vi "GuardarColor.vi"(0 "NombreOperario":string, 3 "TokenColor":T1) -> (5 "HistorialDeColoresOutput":string[](array[string]), 6 "Total De Fichas":dbl, 7 "White":dbl, 9 "Blue":dbl, 10 "Red":dbl)   [LabVIEW 2017]
uses:
  Control/EnumControl.ctl
  Control/ColorTypeEnum.ctl
panel:
  out "Error":string
  out "Verificate2Times":bool
  out "Historial de colores":dbl[](array[numeric])
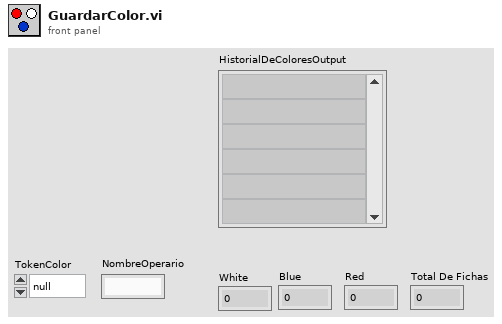
[diagram p1: front panel]
types:
  T1 = typedef "ColorTypeEnum.ctl" = enum16{"null", "White", "Blue", "Red"}
  T2 = typedef "EnumControl.ctl" = enum16{"Default", "Mostrar", "Guardar", "Reiniciar", "Stop", "Error"}
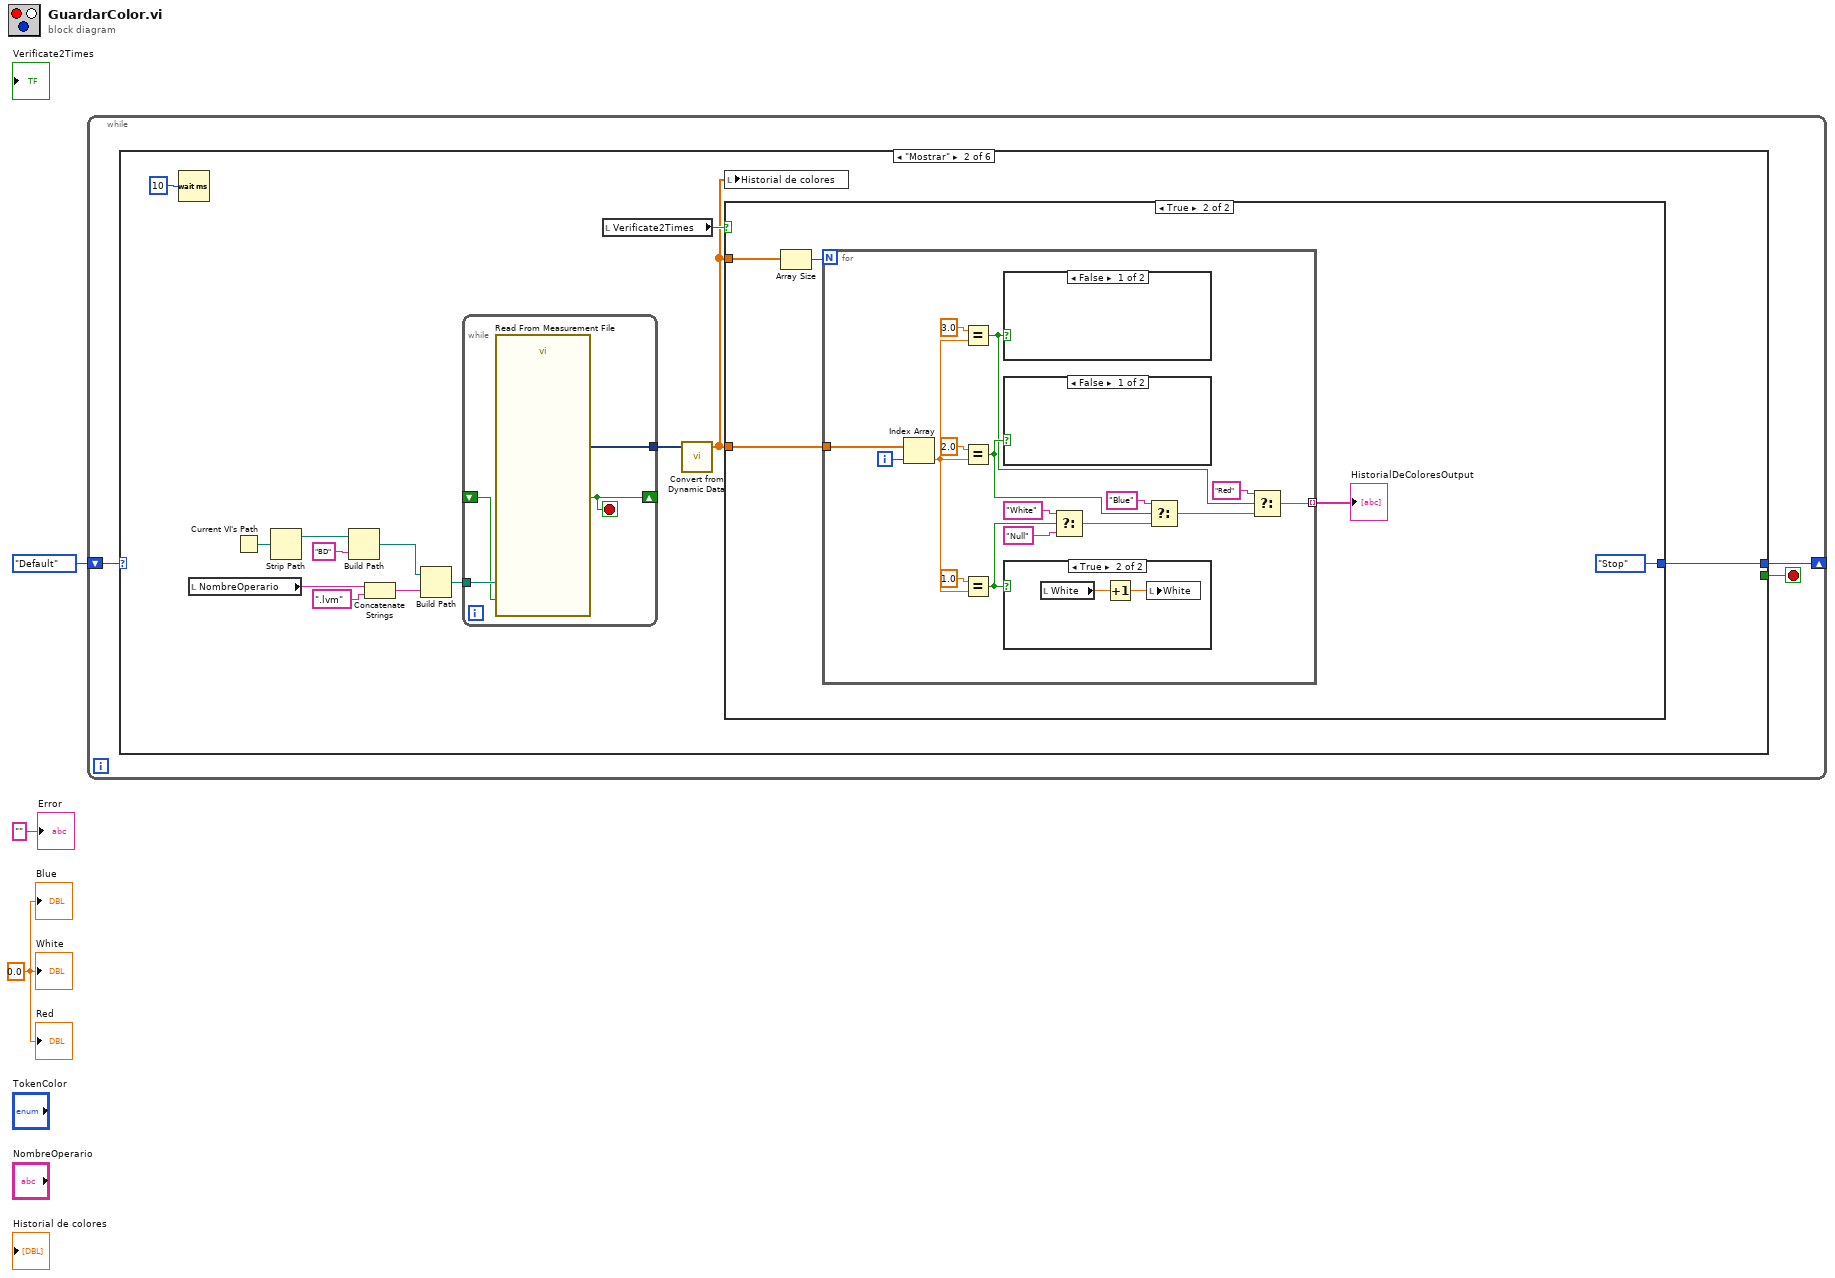
[diagram p0: block diagram]
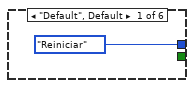
[diagram p2: hidden frame]
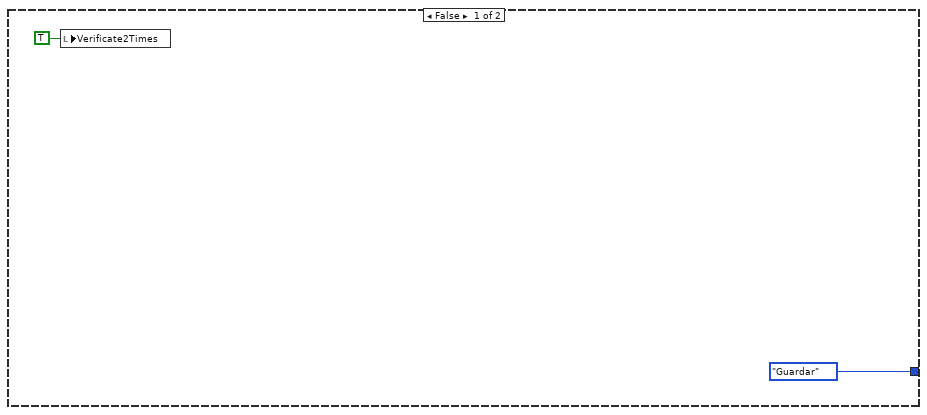
[diagram p3: hidden frame]
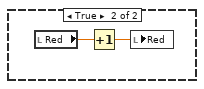
[diagram p5: hidden frame]
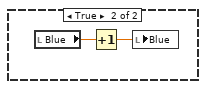
[diagram p6: hidden frame]
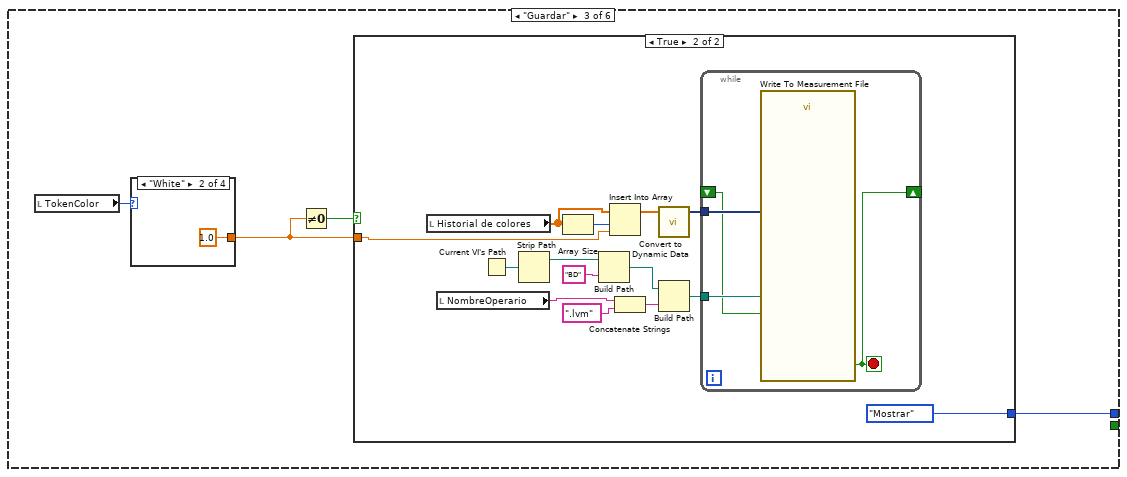
[diagram p7: hidden frame]
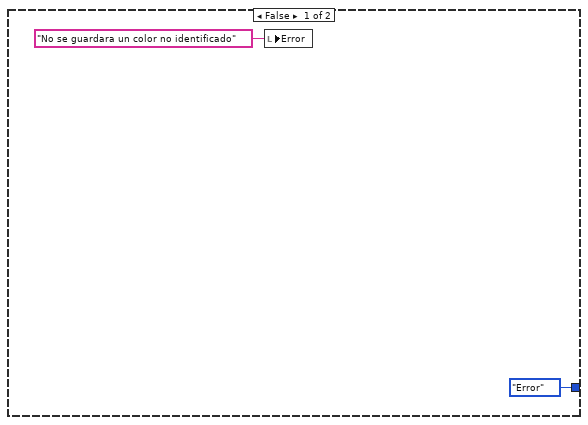
[diagram p8: hidden frame]
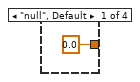
[diagram p9: hidden frame]
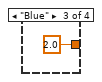
[diagram p10: hidden frame]
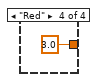
[diagram p11: hidden frame]
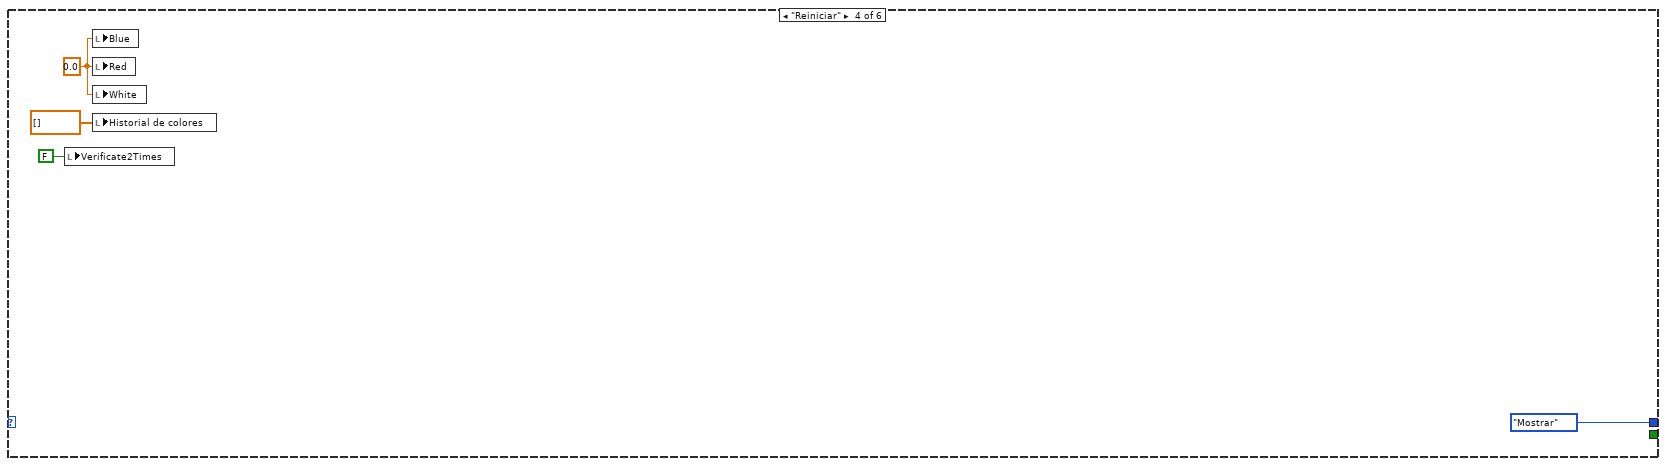
[diagram p12: hidden frame]
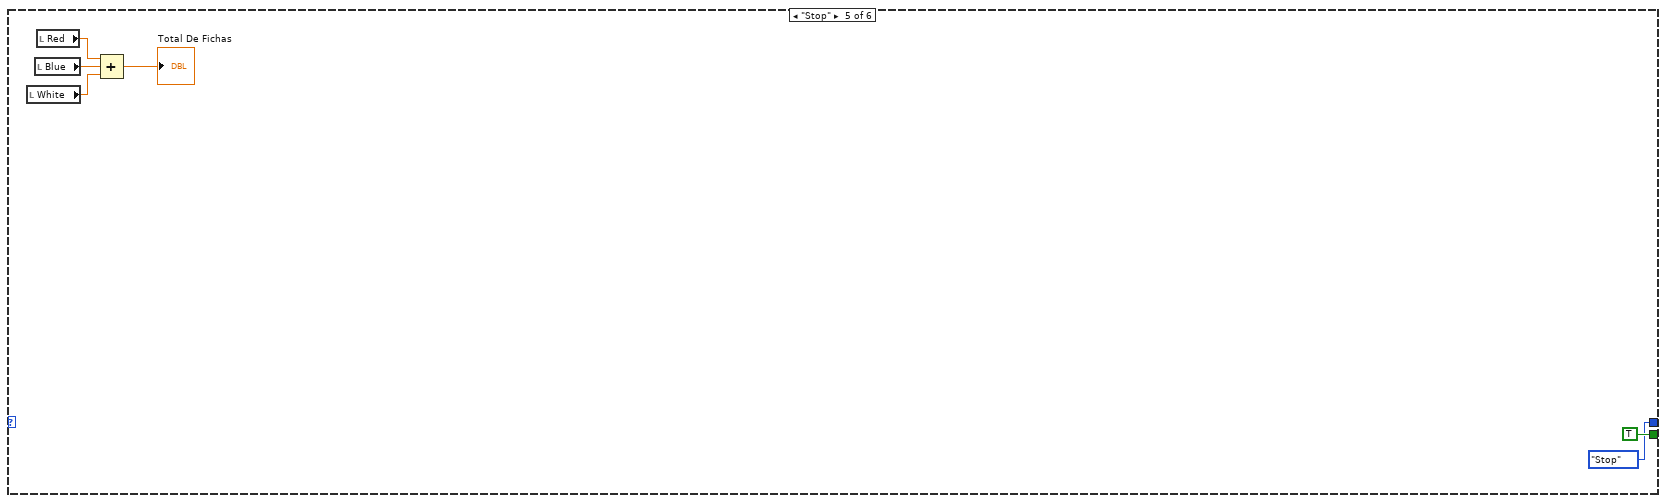
[diagram p13: hidden frame]
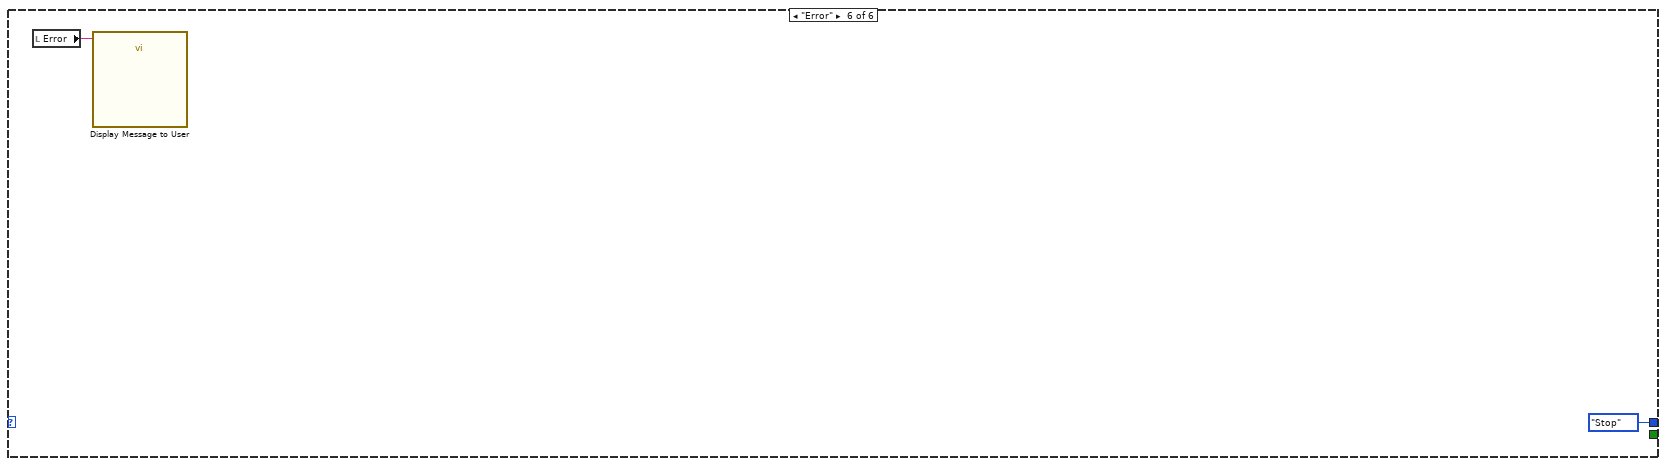
[diagram p14: hidden frame]
diagram:
  w2 = 0.0 ("White")
  n1 = while {
    shift-right: [w4] -> _
    shift-left: EnumControl."Default" -> [w6]
    stop <- w5 stop-if-true
    n2 = case shown="\"Mostrar\"" w6 {
      tunnel: [_ _ _ _ TRUE _] -> w5
      tunnel: [EnumControl."Reiniciar" w10 w54 EnumControl."Mostrar" EnumControl."Stop" EnumControl."Stop"] -> w4
      frame "Default", Default {
      }
      frame "Mostrar" {
        n3 = Wait (ms)(milliseconds to wait=u32 10) -> ()  [unwired: 1 out]
        n4 = local read "NombreOperario"() -> (w11:string)
        n5 = Current VI's Path() -> (path=w14:path)
        n6 = Strip Path(path=w14) -> (stripped path=w17:path)  [unwired: 1 out]
        n7 = Build Path(base path=w17, name or relative path="BD") -> (appended path=w16:path)
        n8 = Concatenate Strings(w11, ".lvm" ("string")) -> (w12:string)
        n9 = Build Path(base path=w16, name or relative path=w12) -> (appended path=w18:path)
        n10 = while {
          tunnel: w18 -> [w53]
          tunnel: [w52] -> w15
          shift-right: [w50] -> _
          shift-left: _ -> [w51]
          stop <- w50 stop-if-true
          n11 = call "Read From Measurement File"("Filename"=w53, "Reset"=w51) -> ("Signals"=w52:dynamicdata, "EOF?"=w50:bool)  [unwired: 4 in, 4 out]
        }
        n12 = local read "Verificate2Times"() -> (w9:bool)
        n13 = call "Convert from Dynamic Data"("Dynamic Data Type"=w15) -> ("Array"=w8:dbl[])  [unwired: 3 in]
        n14 = local write "Historial de colores"(w8) -> ()
        n15 = case shown="True" w9 {
          tunnel: [EnumControl."Guardar" EnumControl."Stop"] -> w10
          tunnel: w8 -> [_ w24]
          tunnel: w8 -> [_ w23]
          frame False {
            n16 = local write "Verificate2Times"(TRUE ("Verificate2Times")) -> ()
          }
          frame True {
            n17 = Array Size(array=w23) -> (size(s)=w25:i32)
            n18 = for {
              N: w25 -> [_]
              tunnel: w24 -> [w43]
              tunnel: [w31] -> w26 mode=indexing
              i -> [w42]
              n19 = Index Array(array=w43, index=w42) -> (element=w36:dbl)
              n20 = Equal?(x=3.0, y=w36) -> (x = y?=w28:bool)
              n21 = Equal?(x=2.0, y=w36) -> (x = y?=w29:bool)
              n22 = Equal?(x=1.0, y=w36) -> (x = y?=w30:bool)
              n23 = case shown="False" w28 {
                frame False {
                }
                frame True {
                  n24 = local read "Red"() -> (w47:dbl)
                  n25 = Increment(x=w47) -> (x+1=w46:dbl)
                  n26 = local write "Red"(w46) -> ()
                }
              }
              n27 = case shown="False" w29 {
                frame False {
                }
                frame True {
                  n28 = local read "Blue"() -> (w49:dbl)
                  n29 = Increment(x=w49) -> (x+1=w48:dbl)
                  n30 = local write "Blue"(w48) -> ()
                }
              }
              n31 = case shown="True" w30 {
                frame False {
                }
                frame True {
                  n32 = local read "White"() -> (w45:dbl)
                  n33 = Increment(x=w45) -> (x+1=w44:dbl)
                  n34 = local write "White"(w44) -> ()
                }
              }
              n35 = Select(t="White", s=w30, f="Null") -> (s? t:f=w35:string)
              n36 = Select(t="Blue", s=w29, f=w35) -> (s? t:f=w33:string)
              n37 = Select(t="Red", s=w28, f=w33) -> (s? t:f=w31:string)
            }
            "HistorialDeColoresOutput" <- w26
          }
        }
      }
      frame "Guardar" {
        n38 = local read "TokenColor"() -> (w57:T1)
        n39 = case shown="\"White\"" w57 {
          tunnel: [0.0 ("new element/subarray") 1.0 ("new element/subarray") 2.0 ("new element/subarray") 3.0 ("new element/subarray")] -> w55
          frame "null", Default {
          }
          frame "White" {
          }
          frame "Blue" {
          }
          frame "Red" {
          }
        }
        n40 = Not Equal To 0?(x=w55) -> (x != 0?=w56:bool)
        n41 = case shown="True" w56 {
          tunnel: w55 -> [_ w61]
          tunnel: [EnumControl."Error" EnumControl."Mostrar"] -> w54
          frame False {
            n42 = local write "Error"("No se guardara un color no identificado" ("Error")) -> ()
          }
          frame True {
            n43 = local read "Historial de colores"() -> (w63:dbl[])
            n44 = local read "NombreOperario"() -> (w62:string)
            n45 = Current VI's Path() -> (path=w68:path)
            n46 = Strip Path(path=w68) -> (stripped path=w73:path)  [unwired: 1 out]
            n47 = Array Size(array=w63) -> (size(s)=w65:i32)
            n48 = Build Path(base path=w73, name or relative path="BD") -> (appended path=w72:path)
            n49 = Insert Into Array(array=w63, index=w65, new element=w61) -> (w66:dbl[])
            n50 = Concatenate Strings(w62, ".lvm" ("string")) -> (w70:string)
            n51 = call "Convert to Dynamic Data"("Array"=w66) -> ("Dynamic Data Type"=w67:dynamicdata)  [unwired: 3 in]
            n52 = Build Path(base path=w72, name or relative path=w70) -> (appended path=w64:path)
            n53 = while {
              tunnel: w67 -> [w77]
              tunnel: w64 -> [w76]
              shift-right: [w75] -> _
              shift-left: _ -> [w74]
              stop <- w75 stop-if-true
              n54 = call "Write To Measurement File"("Signals"=w77, "Reset"=w74, "Filename"=w76) -> ("Saving Data"=w75:bool)  [unwired: 14 in, 2 out]
            }
          }
        }
      }
      frame "Reiniciar" {
        w83 = 0.0 ("Blue")
        n55 = local write "Verificate2Times"(FALSE ("Verificate2Times")) -> ()
        n56 = local write "Blue"(w83) -> ()
        n57 = local write "Red"(w83) -> ()
        n58 = local write "White"(w83) -> ()
        n59 = local write "Historial de colores"(dbl[] [] ("Historial de colores")) -> ()
      }
      frame "Stop" {
        n60 = local read "White"() -> (w87:dbl)
        n61 = local read "Blue"() -> (w88:dbl)
        n62 = local read "Red"() -> (w89:dbl)
        n63 = Compound Arithmetic op=ADD(w89, w88, w87) -> (→"Total De Fichas":dbl)
      }
      frame "Error" {
        n64 = local read "Error"() -> (w92:string)
        n65 = call "Display Message to User"("Message"=w92) -> ()  [unwired: 9 in, 2 out]
      }
    }
  }
  "Blue" <- w2
  "Red" <- w2
  "White" <- w2
  "Error" <- "" ("Error")
